vi "SMD7615 UDP Move.vi"(0 "connection ID in":refnum<k16>, 1 "Acceleration":i32, 2 "Deceleration":i32, 5 "IP":string="192.168.1.30", 7 "Distance / Position":i32, 9 "Velocity":i32, 11 "error in (no error)":errorcluster) -> (4 "connection ID out":refnum<k16>, 15 "error out":errorcluster)   [LabVIEW 2016, in "SMD-7615.lvlib" / "eSCL.lvlib"]
uses:
  eSCL.lvlib
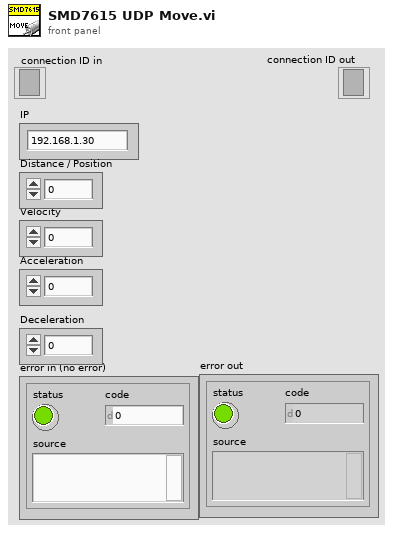
[diagram p1: front panel]
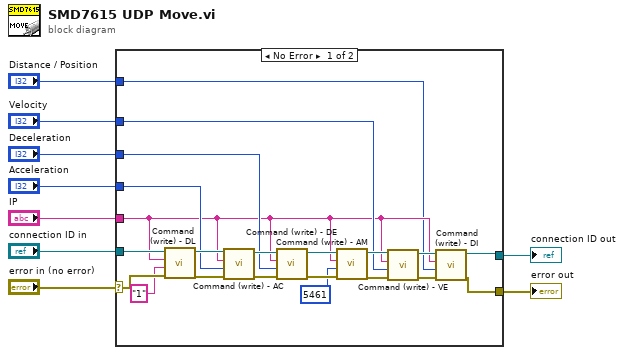
[diagram p0: block diagram]
diagram:
  n1 = case shown="No Error" "error in (no error)" {
    selector: "error in (no error)" -> [w29 w31]
    tunnel: "connection ID in" -> [w30 w32]
    tunnel: [w15 w32] -> w7
    tunnel: [w14 w31] -> w6
    tunnel: "IP" -> [w12 _]
    tunnel: "Acceleration" -> [w25 _]
    tunnel: "Deceleration" -> [w22 _]
    tunnel: "Velocity" -> [w16 _]
    tunnel: "Distance / Position" -> [w10 _]
    frame No Error {
      n2 = call "Command (write) - DL.vi"("error in (no error)"=w29, "Parameter"="1", "IP"=w12, "connection ID in"=w30) -> ("error out"=w26:errorcluster, "connection ID out"=w27:refnum<k16>)  [unwired: 6 in]
      n3 = call "Command (write) - AC.vi"("error in (no error)"=w26, "Acceleration"=w25, "IP"=w12, "connection ID in"=w27) -> ("error out"=w24:errorcluster, "connection ID out"=w23:refnum<k16>)  [unwired: 6 in]
      n4 = call "Command (write) - DE.vi"("error in (no error)"=w24, "Deceleration"=w22, "IP"=w12, "connection ID in"=w23) -> ("error out"=w20:errorcluster, "connection ID out"=w21:refnum<k16>)  [unwired: 6 in]
      n5 = call "Command (write) - AM.vi"("error in (no error)"=w20, "Max. Acceleration"=5461, "IP"=w12, "connection ID in"=w21) -> ("error out"=w17:errorcluster, "connection ID out"=w18:refnum<k16>)  [unwired: 6 in]
      n6 = call "Command (write) - VE.vi"("error in (no error)"=w17, "Velocity"=w16, "IP"=w12, "connection ID in"=w18) -> ("error out"=w11:errorcluster, "connection ID out"=w13:refnum<k16>)  [unwired: 6 in]
      n7 = call "Command (write) - DI.vi"("error in (no error)"=w11, "Distance / Position"=w10, "IP"=w12, "connection ID in"=w13) -> ("error out"=w14:errorcluster, "connection ID out"=w15:refnum<k16>)  [unwired: 6 in]
    }
    frame Error {
    }
  }
  "connection ID out" <- w7
  "error out" <- w6
